vi "Start&Stop_Trigger_2.vi"(11 "TriggerSn":bool) -> (0 "Stop_Tn":u32, 1 "Start_Tn":u32, 4 "Stop_Tn_prev":u32, 5 "TriggerSn_prev0":bool, 6 "Start_Tn_prev":u32, 7 "TriggerSn_prev-1":bool)   [LabVIEW 2020]
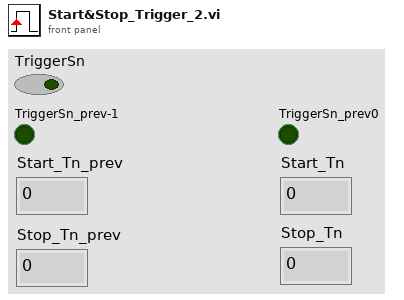
[diagram p1: front panel]
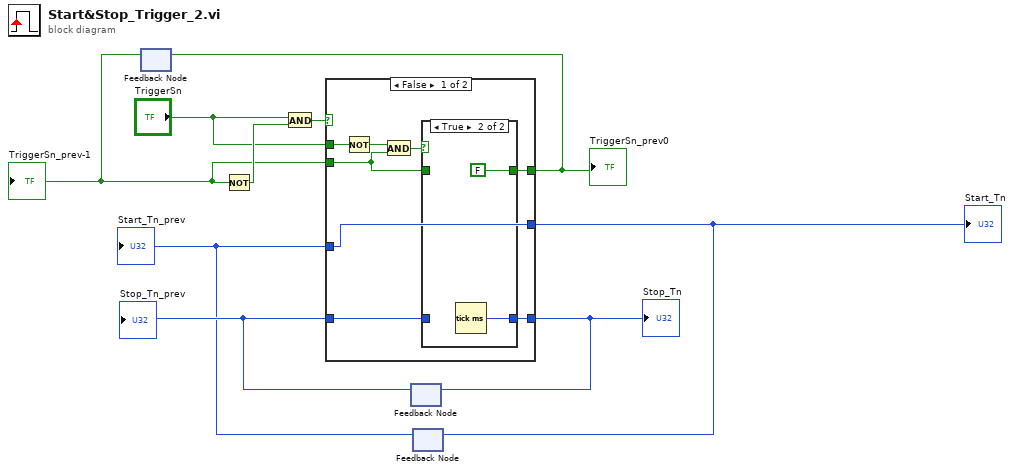
[diagram p0: block diagram]
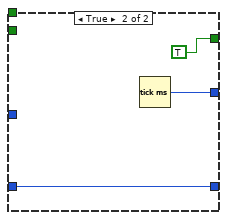
[diagram p3: hidden frame]
diagram:
  n1 = feedback #1() -> (w6:bool)  [unwired: 1 in]
  "TriggerSn_prev-1" <- w6
  n2 = Not(x=w6) -> (.not. x?=w9:bool)
  n3 = And(x="TriggerSn", y=w9) -> (x .and. y?=w8:bool)
  n4 = feedback #2() -> (w3:u32)  [unwired: 1 in]
  "Stop_Tn_prev" <- w3
  n5 = feedback #3() -> (w2:u32)  [unwired: 1 in]
  "Start_Tn_prev" <- w2
  n6 = case shown="False" w8 {
    tunnel: [w17 w24] -> w1
    tunnel: [w12 TRUE] -> w5
    tunnel: w2 -> [w17 _]
    tunnel: w3 -> [w10 w22]
    tunnel: [w13 w22] -> w4
    tunnel: "TriggerSn" -> [w16 _]
    tunnel: w6 -> [w11 _]
    frame False {
      n7 = Not(x=w16) -> (.not. x?=w15:bool)
      n8 = And(x=w15, y=w11) -> (x .and. y?=w14:bool)
      n9 = case shown="True" w14 {
        tunnel: [w18 w21] -> w13
        tunnel: [w19 FALSE] -> w12
        tunnel: w11 -> [w19 _]
        tunnel: w10 -> [w18 _]
        frame False {
        }
        frame True {
          n10 = Tick Count (ms)() -> (millisecond timer value=w21:u32)
        }
      }
    }
    frame True {
      n11 = Tick Count (ms)() -> (millisecond timer value=w24:u32)
    }
  }
  "Start_Tn" <- w1
  "Stop_Tn" <- w4
  "TriggerSn_prev0" <- w5
  n12 = feedback-in #1(w5) -> ()
  n13 = feedback-in #2(w4) -> ()
  n14 = feedback-in #3(w1) -> ()
